vi "Search BuildSpec Tags.vi"(8 "error in (no error)":errorcluster, 10 "Regular expression":string="Bld_excludedDirectory", 11 "BuildSpec in":refnum<vi>) -> (0 "error out":errorcluster, 2 "Tag Names":string[](array[string]), 3 "BuildSpec out":refnum<vi>)   [LabVIEW 2019, in "Project Sync Tools.lvclass"]
uses:
  Project Sync Tools.lvclass
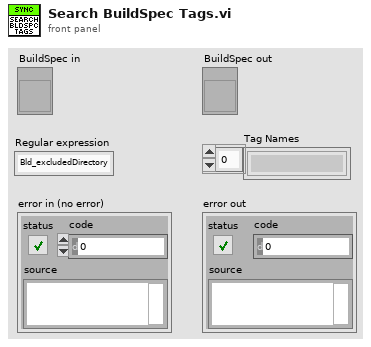
[diagram p1: front panel]
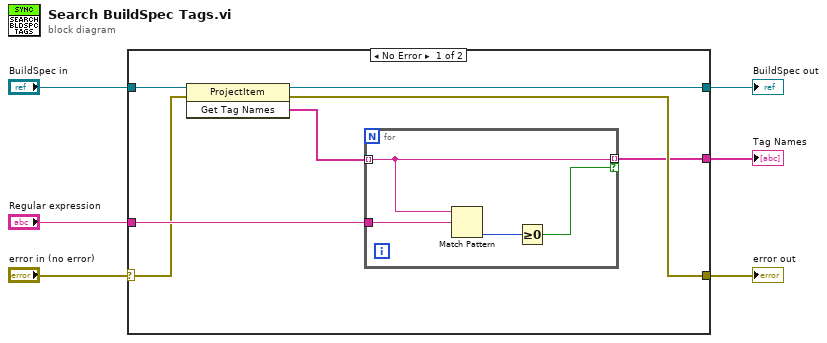
[diagram p0: block diagram]
diagram:
  n1 = case shown="No Error" "error in (no error)" {
    selector: "error in (no error)" -> [w7 w18]
    tunnel: [w13 w18] -> w6
    tunnel: [w12 w19] -> w5
    tunnel: "BuildSpec in" -> [w11 w19]
    tunnel: [w10 _] -> w3
    tunnel: "Regular expression" -> [w9 _]
    frame No Error {
      n2 = invoke class="ProjectItem" method="Get Tag Names"(reference=w11, error in=w7) -> (reference out=w12:refnum<vi>, error out=w13:errorcluster, "Get Tag Names"=w8:string[])  [unwired: 1 in]
      n3 = for {
        tunnel: w8 -> [w15] mode=indexing
        tunnel: w9 -> [w17]
        tunnel: [w15] -> w10 mode=indexing if=w14
        n4 = Match Pattern(string=w15, regular expression=w17) -> (offset past match=w16:i32)  [unwired: 1 in, 3 out]
        n5 = Greater Or Equal To 0?(x=w16) -> (x >= 0?=w14:bool)
      }
    }
    frame Error {
    }
  }
  "error out" <- w6
  "BuildSpec out" <- w5
  "Tag Names" <- w3
